vi "E4351B_main_2s1p.vi"() -> ()   [LabVIEW 2016]
doc: "Programs an SAS list for channel 1, set the transient trigger to increment it continuously, and set the data logger to take continuous measurements of channel 1's output. Finally, channel 1's voltage and curent outputs are displayed using charts."
uses:
  <vilib>/Utility/file.llb/Read Delimited Spreadsheet (DBL).vi
  <instrlib>/Agilent E4351B/Agilent E4351B.lvlib
panel:
  in  "file path":path=path "C:/Software_Repository/BDC_prototype/logger/toVI_sec.csv"
  out "XY Graph":cluster{dbl[], dbl[]}(graph)
  out "Numeric":dbl
  out "Current":cluster{dbl[], dbl[]}(graph)
  out "Voltage":cluster{dbl[], dbl[]}(graph)
  in  "Stop VI":bool
  in  "VISA resource name":refnum<visa-resource-name>="GPIB0::2::INSTR"
  # "(c) CHANGED TOO MUCH"
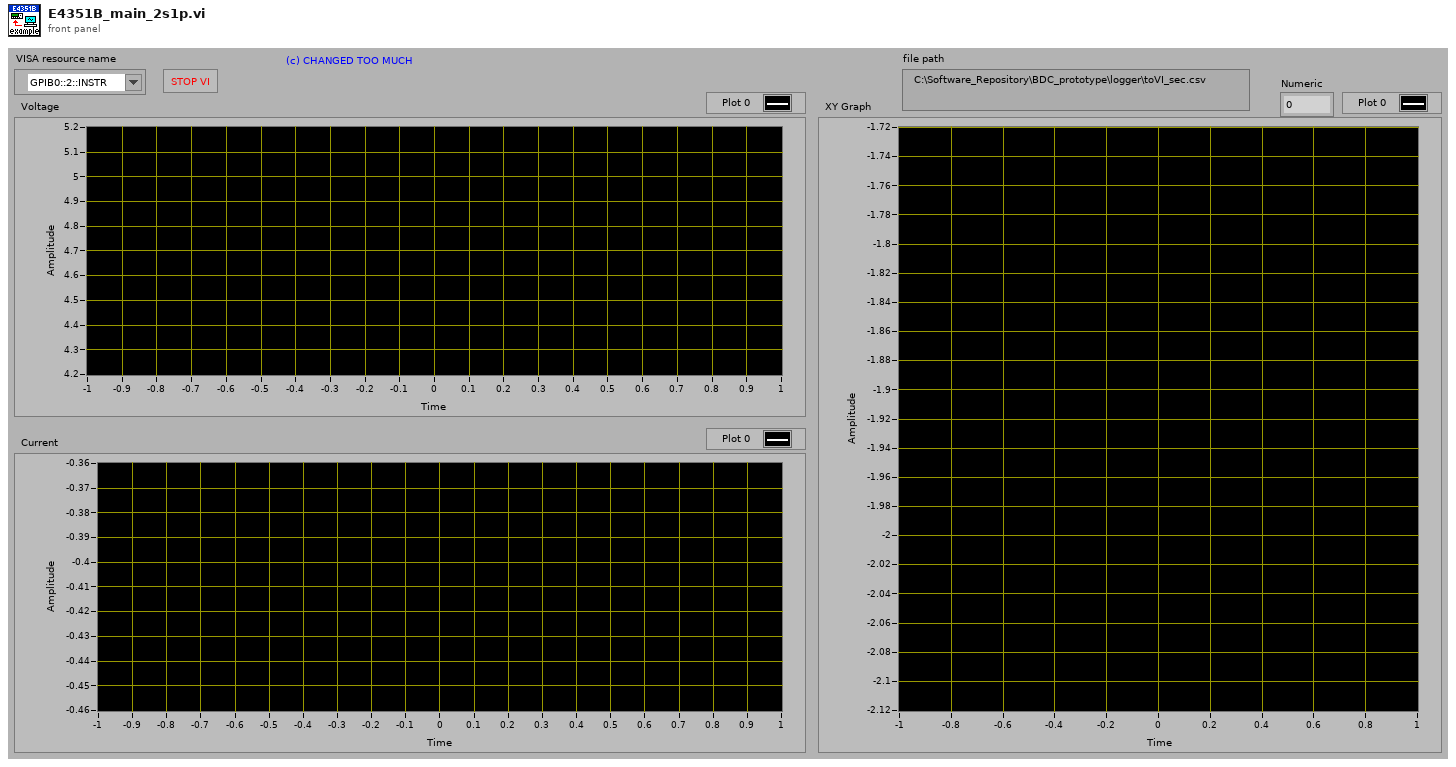
[diagram p1: front panel]
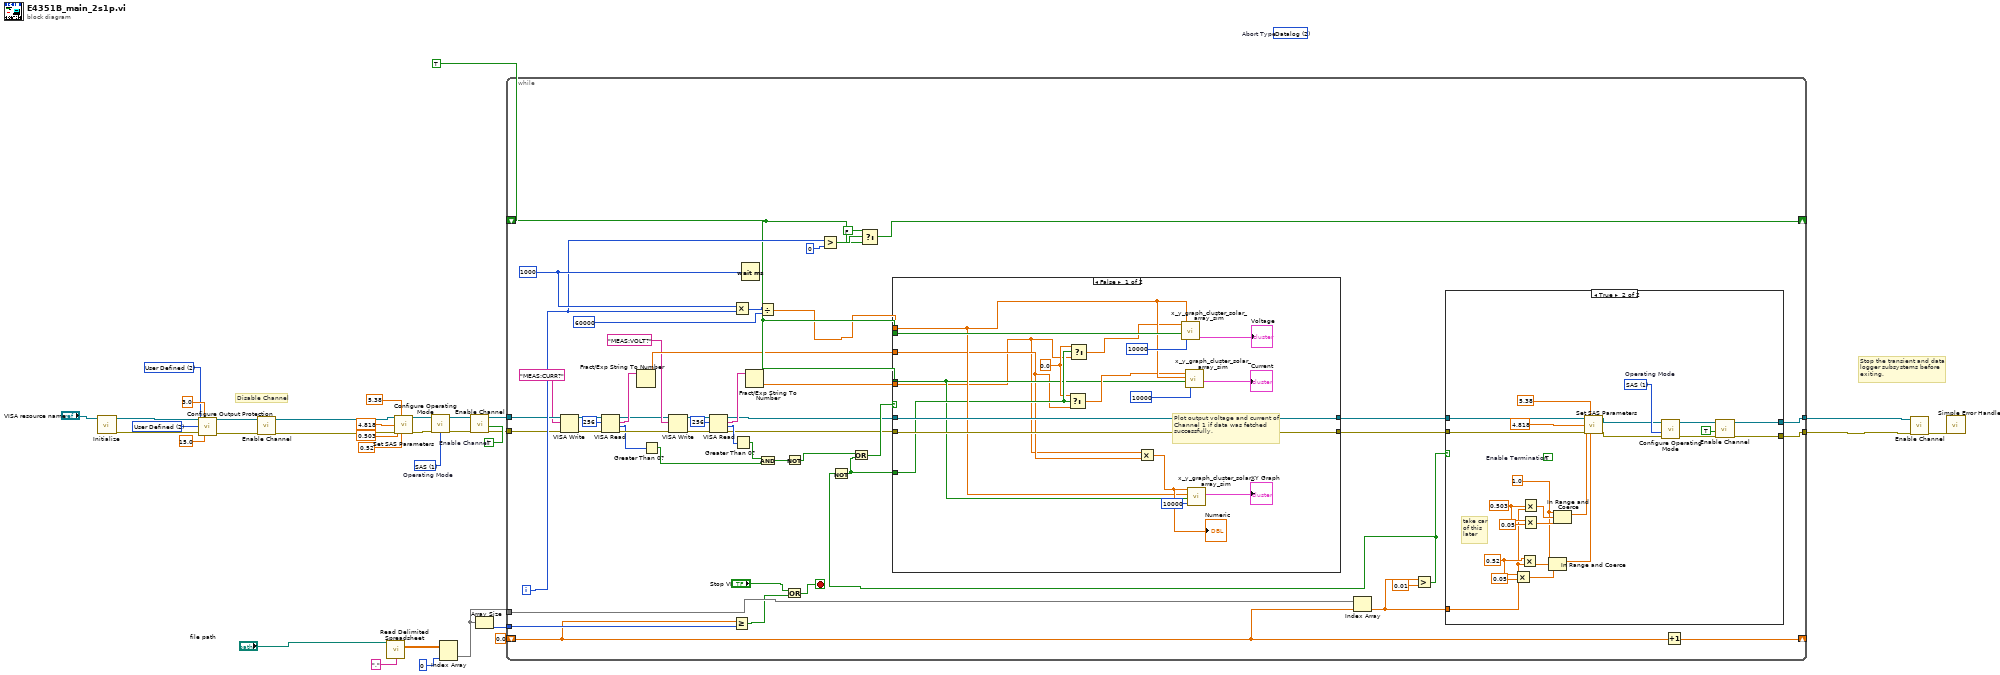
[diagram p0: block diagram]
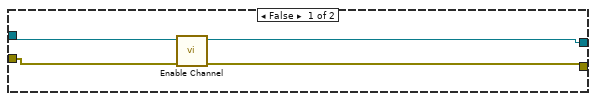
[diagram p2: hidden frame]
diagram:
  w26 = 2 items=["MAX", "MIN", "User Defined"] ("Voltage Limit Source (0:MAX)")
  w27 = 2 items=["MAX", "MIN", "User Defined"] ("Current Limit Source (0:MAX)")
  w32 = TRUE  # Enable Channel
  (unwired) 2 items=["Transient", "Acquire", "Datalog"]  # Abort Type
  w33 = 1 items=["Fixed", "SAS", "Table"]  # Operating Mode
  # "Disable Channel"
  # "Stop the transient and data logger subsystems before exiting."
  n1 = call <instrlib>:"Initialize.vi"("VISA resource name"="VISA resource name") -> ("error out"=w30:errorcluster, "VISA resource name out"=w31:refnum<visa-resource-name>)  [unwired: 9 in]
  n2 = call <instrlib>:"Configure Output Protection.vi"("VISA resource name"=w31, "Current Limit (0 A)"=3.0, "Current Limit Source (0:MAX)"=w27, "Voltage Limit Source (0:MAX)"=w26, "error in (no error)"=w30, "Voltage Limit (0 V)"=15.0) -> ("VISA resource name out"=w9:refnum<visa-resource-name>, "error out"=w8:errorcluster)  [unwired: 8 in]
  n3 = call <instrlib>:"Enable Channel.vi"("error in (no error)"=w8, "VISA resource name"=w9) -> ("error out"=w24:errorcluster, "VISA resource name out"=w25:refnum<visa-resource-name>)  [unwired: 8 in]
  n4 = call-poly <vilib>:"Read Delimited Spreadsheet.vi"("file path (dialog if empty)"="file path", "delimiter (\\t)"="," ("delimiter (\\t)")) -> ("all rows"=w12:dbl[][])  [unwired: 8 in, 5 out]
  n5 = call <instrlib>:"Set SAS Parameters.vi"("VISA resource name"=w25, "Open Circuit Voltage (0.0 V)"=5.38, "Maximum Voltage Point (0.0 V)"=4.818, "Maximum Current Point (0.0 A)"=0.503, "error in (no error)"=w24, "Short Circuit Current (0.0 A)"=0.52) -> ("VISA resource name out"=w17:refnum<visa-resource-name>, "error out"=w16:errorcluster)  [unwired: 8 in]
  n6 = call <instrlib>:"Configure Operating Mode.vi"("error in (no error)"=w16, "Operating Mode (0:Fixed)"=w33, "VISA resource name"=w17) -> ("error out"=w6:errorcluster, "VISA resource name out"=w7:refnum<visa-resource-name>)  [unwired: 7 in]
  n7 = Index Array(array=w12, index (col)=0 ("disabled index (col)")) -> (element=w11:dbl[])  [unwired: 1 in]
  n8 = call <instrlib>:"Enable Channel.vi"("error in (no error)"=w6, "Enable Channel (Disable)"=w32, "VISA resource name"=w7) -> ("error out"=w4:errorcluster, "VISA resource name out"=w5:refnum<visa-resource-name>)  [unwired: 7 in]
  n9 = Array Size(array=w11) -> (size(s)=w10:i32)
  n10 = while {
    tunnel: w5 -> [w59]
    tunnel: [w72] -> w3
    shift-right: [w81] -> _
    shift-left: TRUE -> [w76]
    tunnel: [w71] -> w2
    shift-right: [w73] -> _
    shift-left: 0.0 -> [w35]
    tunnel: w4 -> [w58]
    tunnel: w11 -> [w70]
    tunnel: w10 -> [w67]
    i -> [w80]
    stop <- w65 stop-if-true
    w84 = u32 1000 ("milliseconds to wait")
    n11 = VISA Write(VISA resource name=w59, write buffer="MEAS:CURR?", error in (no error)=w58) -> (VISA resource name out=w55:refnum<visa-resource-name>, error out=w56:errorcluster)  [unwired: 1 out]
    n12 = VISA Read(VISA resource name=w55, byte count=u32 256, error in (no error)=w56) -> (VISA resource name out=w46:refnum<visa-resource-name>, read buffer=w53:string, return count=w42:u32, error out=w45:errorcluster)
    n13 = Fract/Exp String To Number(string=w53) -> (number=w52:dbl)  [unwired: 3 in, 1 out]
    n14 = Greater Than 0?(x=w42) -> (x > 0?=w40:bool)
    n15 = VISA Write(VISA resource name=w46, write buffer="MEAS:VOLT?", error in (no error)=w45) -> (VISA resource name out=w49:refnum<visa-resource-name>, error out=w50:errorcluster)  [unwired: 1 out]
    n16 = VISA Read(VISA resource name=w49, byte count=u32 256, error in (no error)=w50) -> (VISA resource name out=w39:refnum<visa-resource-name>, read buffer=w47:string, return count=w43:u32, error out=w38:errorcluster)
    n17 = Greater Or Equal?(x=w35, y=w67) -> (x >= y?=w64:bool)
    n18 = Multiply(x=w84, y=w80) -> (x*y=w83:u32)
    n19 = Greater Than 0?(x=w43) -> (x > 0?=w41:bool)
    n20 = Wait (ms)(milliseconds to wait=w84) -> ()  [unwired: 1 out]
    n21 = Fract/Exp String To Number(string=w47) -> (number=w44:dbl)  [unwired: 3 in, 1 out]
    n22 = Divide(x=w83, y=u32 60000) -> (x/y=w63:dbl)
    n23 = And(x=w41, y=w40) -> (x .and. y?=w37:bool)
    n24 = Not(x=w37) -> (.not. x?=w36:bool)
    n25 = Or(x="Stop VI", y=w64) -> (x .or. y?=w65:bool)
    n26 = Greater?(x=w80, y=0) -> (0:w78:bool)
    n27 = Select(t=FALSE, s=w78, f=w76) -> (s? t:f=w81:bool)
    n28 = Index Array(array=w70, index=w35) -> (element=w69:dbl)
    n29 = Greater?(x=w69, y=0.01) -> (0:w61:bool)
    n30 = Not(x=w61) -> (.not. x?=w60:bool)
    n31 = Or(x=w36, y=w60) -> (x .or. y?=w62:bool)
    n32 = case shown="False" w62 {
      tunnel: [w130 w132] -> w75
      tunnel: w39 -> [w130 w132]
      tunnel: w38 -> [w129 w131]
      tunnel: [w129 w131] -> w74
      tunnel: w63 -> [w122 _]
      tunnel: w76 -> [w124 _]
      tunnel: w76 -> [w115 _]
      tunnel: w60 -> [w117 _]
      tunnel: w52 -> [w114 _]
      tunnel: w44 -> [w113 _]
      frame False {
        w116 = 0.0 ("t")
        # "Plot output voltage and current of Channel 1 if data was fetched successfully."
        n33 = Select(t=w116, s=w117, f=w114) -> (s? t:f=w119:dbl)
        n34 = Select(t=w116, s=w117, f=w113) -> (s? t:f=w118:dbl)
        n35 = Multiply(x=w113, y=w114) -> (x*y=w123:dbl)
        "Numeric" <- w123
        n36 = call "x_y_graph_cluster_solar_array_sim.vi"("Chart History (10,000)"=10000, "Clear Graph?"=w124, "X"=w122, "Y"=w118) -> ("Cluster"=→"Voltage":cluster{dbl[], dbl[]})
        n37 = call "x_y_graph_cluster_solar_array_sim.vi"("Chart History (10,000)"=10000, "Clear Graph?"=w115, "X"=w122, "Y"=w119) -> ("Cluster"=→"Current":cluster{dbl[], dbl[]})
        n38 = call "x_y_graph_cluster_solar_array_sim.vi"("Chart History (10,000)"=10000, "Clear Graph?"=w115, "X"=w122, "Y"=w123) -> ("Cluster"=→"XY Graph":cluster{dbl[], dbl[]})
      }
      frame True {
      }
    }
    n39 = case shown="True" w61 {
      tunnel: w75 -> [w88 w111]
      tunnel: w74 -> [w86 w110]
      tunnel: [w87 w93] -> w72
      tunnel: [w85 w94] -> w71
      tunnel: w69 -> [_ w97]
      frame False {
        n40 = call <instrlib>:"Enable Channel.vi"("error in (no error)"=w86, "VISA resource name"=w88) -> ("error out"=w85:errorcluster, "VISA resource name out"=w87:refnum<visa-resource-name>)  [unwired: 8 in]
      }
      frame True {
        w89 = 1.0 ("upper limit")
        w100 = 1 items=["Fixed", "SAS", "Table"]  # Operating Mode
        w104 = 0.52 ("Maximum Current Point (0.0 A)")
        w107 = 0.503 ("Maximum Current Point (0.0 A)")
        (unwired) TRUE  # Enable Termination
        # "take car\nof this \nlater"
        n41 = Multiply(x=w104, y=0.05) -> (x*y=w102:dbl)
        n42 = Multiply(x=w104, y=w97) -> (x*y=w90:dbl)
        n43 = Multiply(x=w107, y=w97) -> (x*y=w91:dbl)
        n44 = Multiply(x=w107, y=0.05) -> (x*y=w105:dbl)
        n45 = In Range and Coerce(upper limit=w89, x=w90, lower limit=w102) -> (coerced(x)=w101:dbl)  [unwired: 1 out]
        n46 = In Range and Coerce(upper limit=w89, x=w91, lower limit=w105) -> (coerced(x)=w108:dbl)  [unwired: 1 out]
        n47 = call <instrlib>:"Set SAS Parameters.vi"("VISA resource name"=w111, "Open Circuit Voltage (0.0 V)"=5.38, "Maximum Voltage Point (0.0 V)"=4.818, "Maximum Current Point (0.0 A)"=w108, "error in (no error)"=w110, "Short Circuit Current (0.0 A)"=w101) -> ("VISA resource name out"=w99:refnum<visa-resource-name>, "error out"=w98:errorcluster)  [unwired: 8 in]
        n48 = call <instrlib>:"Configure Operating Mode.vi"("error in (no error)"=w98, "Operating Mode (0:Fixed)"=w100, "VISA resource name"=w99) -> ("error out"=w95:errorcluster, "VISA resource name out"=w96:refnum<visa-resource-name>)  [unwired: 7 in]
        n49 = call <instrlib>:"Enable Channel.vi"("error in (no error)"=w95, "Enable Channel (Disable)"=TRUE, "VISA resource name"=w96) -> ("error out"=w94:errorcluster, "VISA resource name out"=w93:refnum<visa-resource-name>)  [unwired: 7 in]
      }
    }
    n50 = Increment(x=w35) -> (x+1=w73:dbl)
  }
  n51 = call <instrlib>:"Enable Channel.vi"("error in (no error)"=w2, "VISA resource name"=w3) -> ("error out"=w1:errorcluster)  [unwired: 8 in, 1 out]
  n52 = call <vilib>:"Simple Error Handler.vi"("error in (no error)"=w1) -> ()  [unwired: 4 in, 5 out]
